vi "Single button press.vi"(11 "Button Value":bool) -> (3 "Button Press":bool)   [LabVIEW 2017]
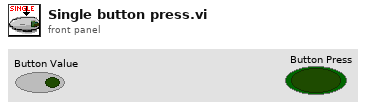
[diagram p1: front panel]
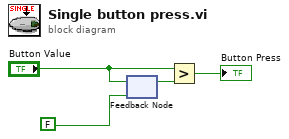
[diagram p0: block diagram]
diagram:
  n1 = feedback #1(FALSE) -> (w4:bool)
  n2 = feedback-in #1("Button Value") -> ()
  n3 = Greater?(x="Button Value", y=w4) -> (0:→"Button Press":bool)
